vi "Wait.vi"(8 "error in (no error)":errorcluster, 11 "Timer in":refnum<class "Timer.lvclass">) -> (0 "error out":errorcluster, 1 "elapsed time(s)":dbl, 2 "timeout":bool, 3 "Timer out":refnum<class "Timer.lvclass">, 4 "pause?":bool)   [LabVIEW 2020, in "Timer.lvclass"]
uses:
  Timer.lvclass
  Timer.lvclass/Timer.ctl
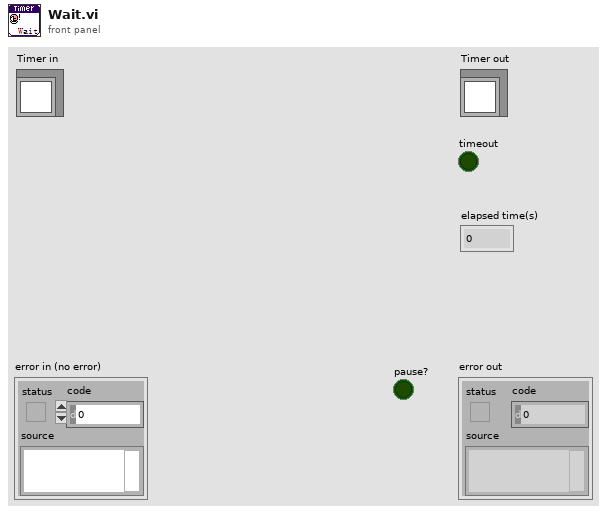
[diagram p1: front panel]
types:
  T1 = cluster{"target time(ms)":u32, "elapsed time(ms)":u32, "start time":u32, "pause":bool, "auto reset":bool}
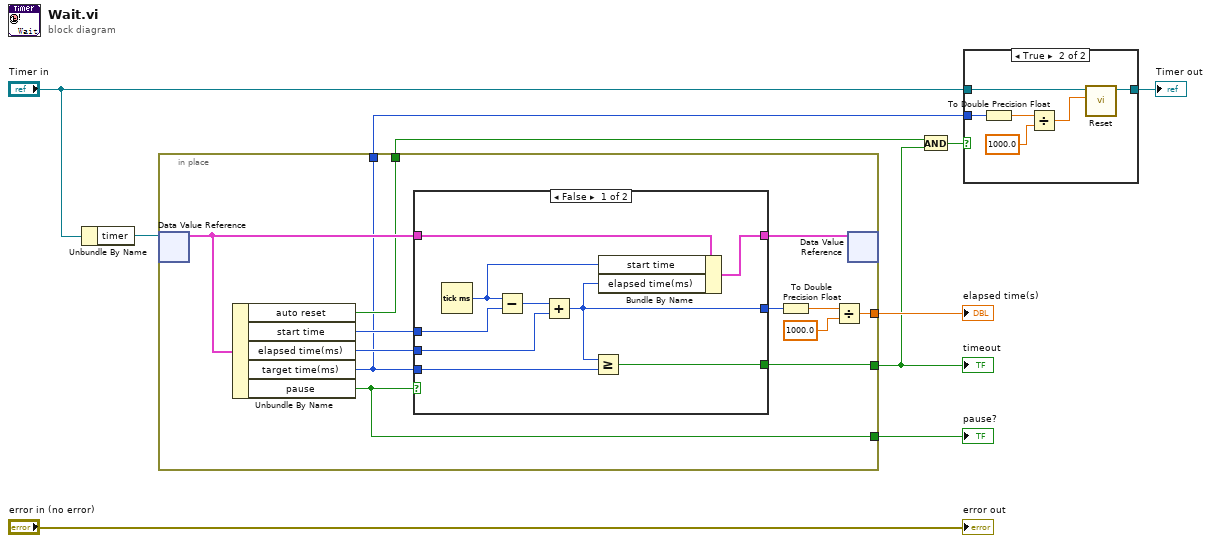
[diagram p0: block diagram]
diagram:
  n1 = Unbundle By Name("Timer in") -> ("timer"=w10:refnum<data-value>)
  n2 = in-place {
    in-place-border: [w19] -> w5
    in-place-border: [w15] -> w9
    in-place-border: [w13] -> w2
    in-place-border: [w12] -> w3
    in-place-border: [w11] -> w1
    n3 = in-place-dvr #1(w10) -> (w22:T1)  [unwired: 1 out]
    n4 = Unbundle By Name(w22) -> ("auto reset"=w13:bool, "start time"=w20:u32, "elapsed time(ms)"=w21:u32, "target time(ms)"=w12:u32, "pause"=w11:bool)
    n5 = case shown="False" w11 {
      tunnel: w20 -> [w31 _]
      tunnel: w21 -> [w25 w32]
      tunnel: [w30 _] -> w19
      tunnel: w12 -> [w24 _]
      tunnel: w22 -> [w29 w33]
      tunnel: [w27 w33] -> w18
      tunnel: [w23 w32] -> w16
      frame False {
        n6 = Tick Count (ms)() -> (millisecond timer value=w28:u32)
        n7 = Subtract(x=w28, y=w31) -> (x-y=w26:u32)
        n8 = Add(x=w26, y=w25) -> (x+y=w23:u32)
        n9 = Greater Or Equal?(x=w23, y=w24) -> (x >= y?=w30:bool)
        n10 = Bundle By Name(cluster=w29, "start time"=w28, "elapsed time(ms)"=w23) -> (w27:T1)
      }
      frame True {
      }
    }
    n11 = To Double Precision Float(number=w16) -> (double precision float=w17:dbl)
    n12 = Divide(x=w17, y=1000.0) -> (x/y=w15:dbl)
    n13 = in-place-dvr #1(w18) -> ()  [unwired: 2 out]
  }
  "timeout" <- w5
  "elapsed time(s)" <- w9
  "pause?" <- w1
  n14 = And(x=w2, y=w5) -> (x .and. y?=w4:bool)
  n15 = case shown="True" w4 {
    tunnel: [w34 w40] -> w7
    tunnel: "Timer in" -> [w34 w39]
    tunnel: w3 -> [_ w38]
    frame False {
    }
    frame True {
      n16 = To Double Precision Float(number=w38) -> (double precision float=w37:dbl)
      n17 = Divide(x=w37, y=1000.0) -> (x/y=w35:dbl)
      n18 = call "Reset.vi"("target time(1s)"=w35, "Timer in"=w39) -> ("Timer out"=w40:refnum<class "Timer.lvclass">)  [unwired: 8 in, 1 out]
    }
  }
  "Timer out" <- w7
  "error out" <- "error in (no error)"
